vi "ADIS16448 Set Calibration Time.vi"(8 "error in (no error)":errorcluster, 10 "Calibration Time":T1, 11 "ADIS16448DevRef in":T2={"DevStatus"={"status"=FALSE, "code"=0, "source"=""}, "Hardware Config"={"SPI Clock Rate (Hz)"=1000000.0, "IMU SPI Mode (3)"=enum."Mode 3 (Clk Idle High,Sample on Trailing)", "IMU Reset Pin"=enum."SPI Port CS2", "IMU SPI Bus"=enum."SPI On-Board, CS0", "IMU Data Ready Pin"=enum."SPI Port CS1", "Stall Config"={"Pow2BytesPerRead"=255, "StallTicks"=640, "CsToSclkTicks"=5}, "IMU Status LED Pin"=enum."DIO MXP 9"}, "Calibration Complete"=refnum, "Status reference"=refnum, "Sychronous Process VI"=refnum, "Cmd FIFO"=refnum, "Source"={"DevStatus"={"status"=FALSE, "code"=0, "source"=""}, "AnalogTriggerMode?"=FALSE, "DigitalMode"={"DIO Channel"=enum."Disabled"}, "AnalogTriggerMode"={"AnalogTriggerIndex"=enum."Trig 0", "OutputType"=enum."InWindow"}}, "Data FIFO"=refnum, "IMU Status LED Pin"=enum."DIO MXP 9", "Calibration Time (ms)"=0, "Data Reference"=refnum}) -> (0 "error out":errorcluster, 3 "ADIS16448DevRef out":T2={"DevStatus"={"status"=FALSE, "code"=0, "source"=""}, "Hardware Config"={"SPI Clock Rate (Hz)"=1000000.0, "IMU SPI Mode (3)"=enum."Mode 3 (Clk Idle High,Sample on Trailing)", "IMU Reset Pin"=enum."SPI Port CS2", "IMU SPI Bus"=enum."SPI On-Board, CS0", "IMU Data Ready Pin"=enum."SPI Port CS1", "Stall Config"={"Pow2BytesPerRead"=255, "StallTicks"=640, "CsToSclkTicks"=5}, "IMU Status LED Pin"=enum."DIO MXP 9"}, "Calibration Complete"=refnum, "Status reference"=refnum, "Sychronous Process VI"=refnum, "Cmd FIFO"=refnum, "Source"={"DevStatus"={"status"=FALSE, "code"=0, "source"=""}, "AnalogTriggerMode?"=FALSE, "DigitalMode"={"DIO Channel"=enum."Disabled"}, "AnalogTriggerMode"={"AnalogTriggerIndex"=enum."Trig 0", "OutputType"=enum."InWindow"}}, "Data FIFO"=refnum, "IMU Status LED Pin"=enum."DIO MXP 9", "Calibration Time (ms)"=0, "Data Reference"=refnum})   [LabVIEW 2025]
doc: "This VI is deprecated. Use the input on the recalibrate VI instead."
uses:
  <vilib>/Rock Robotics/WPI/ThirdParty/ADI/ADIS16448/Typedef/ADIS16448 Command Type.ctl
  <vilib>/Rock Robotics/SystemInterfaces/DIO/FPGA_DIOChannel.ctl
  <vilib>/Rock Robotics/SystemInterfaces/spilib/spi_bus.ctl
  <vilib>/Rock Robotics/WPI/SPI/WPI_SPIMode.ctl
  <vilib>/Rock Robotics/WPI/ThirdParty/ADI/ADIS16448/Typedef/ADIS16448 Hardware Configuration.ctl
  <vilib>/Rock Robotics/WPI/ThirdParty/ADI/ADIS16448/Typedef/ADIS16448 Device Reference.ctl
  <vilib>/Rock Robotics/WPI/ThirdParty/ADI/ADIS16448/Typedef/ADIS16448 Data.ctl
  <vilib>/Rock Robotics/WPI/ThirdParty/ADI/ADIS16448/Typedef/ADIS16448 Status.ctl
  <vilib>/Rock Robotics/WPI/ThirdParty/ADI/ADIS16448/Typedef/ADIS16448 Process.ctl
  <vilib>/Rock Robotics/SystemInterfaces/DIO/FPGA_DIODigitalSourceChannel.ctl
  <vilib>/Rock Robotics/SystemInterfaces/AnalogTrigger/FPGA_AnalogTriggerIndex.ctl
  <vilib>/Rock Robotics/SystemInterfaces/AnalogTrigger/FPGA_AnalogTriggerOutType.ctl
  <vilib>/Rock Robotics/SystemInterfaces/CounterEncoderSourceConvertion/FPGA_CounterEncoderSourceConvertionLVSourceType.ctl
  <vilib>/Rock Robotics/WPI/ThirdParty/ADI/ADIS16448/Typedef/ADIS16448 Calibration Time.ctl
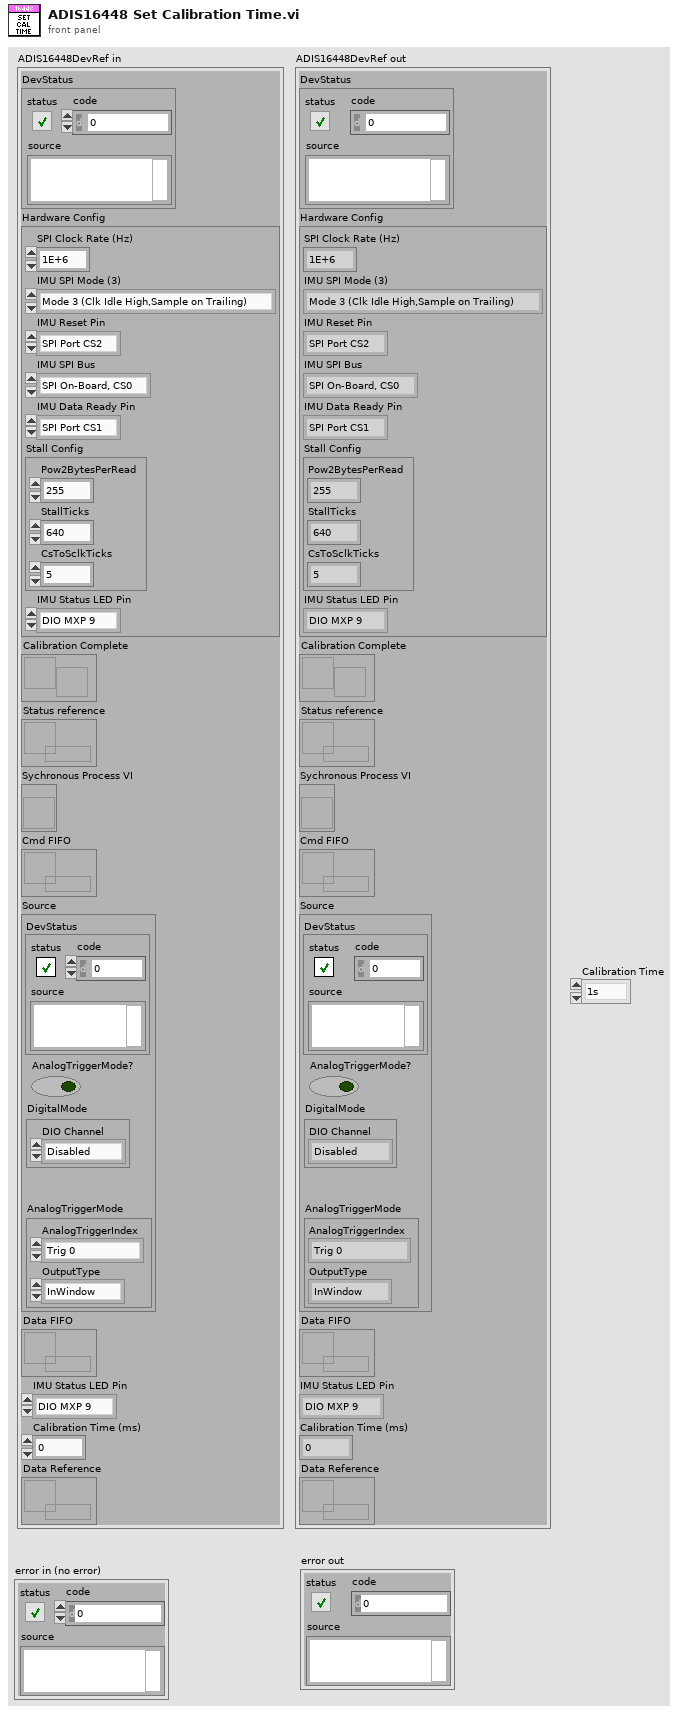
[diagram p1: front panel]
types:
  T1 = typedef "ADIS16448 Calibration Time.ctl" = enum16{"1s", "s", "4.9ms", "9.8ms", "19.5ms", "39.1ms", "78.1ms", "156.3ms", "312.5ms", "625ms", "1.25s", "2.5s", "5s", "10s", "20s", "40s", "80s", "160s", "320s"}
  T2 = typedef "ADIS16448 Device Reference.ctl" = cluster{"DevStatus":errorcluster, "Hardware Config":T3, "Calibration Complete":refnum<notifier>, "Status reference":refnum<data-value>, "Sychronous Process VI":T7, "Cmd FIFO":refnum<k33>, "Source":T8, "Data FIFO":refnum<k33>, "IMU Status LED Pin":T5, "Calibration Time (ms)":u32, "Data Reference":refnum<data-value>}
  T3 = typedef "ADIS16448 Hardware Configuration.ctl" = cluster{"SPI Clock Rate (Hz)":dbl, "IMU SPI Mode (3)":T4, "IMU Reset Pin":T5, "IMU SPI Bus":T6, "IMU Data Ready Pin":T5, "Stall Config":cluster{"Pow2BytesPerRead":u8, "StallTicks":u16, "CsToSclkTicks":u8}, "IMU Status LED Pin":T5}
  T4 = typedef "WPI_SPIMode.ctl" = enum16{"Mode 0 (Clk Idle Low,Sample on Leading)", "Mode 1 (Clk Idle Low,Sample on Trailing)", "Mode 2 (Clk Idle High,Sample on Leading)", "Mode 3 (Clk Idle High,Sample on Trailing)"}
  T5 = typedef "FPGA_DIOChannel.ctl" = enum8{"DIO 0", "DIO 1", "DIO 2", "DIO 3", "DIO 4", "DIO 5", "DIO 6", "DIO 7", "DIO 8", "DIO 9", "DIO MXP 0", "DIO MXP 1", "DIO MXP 2", "DIO MXP 3", "DIO MXP 4", "DIO MXP 5", "DIO MXP 6", "DIO MXP 7", "DIO MXP 8", "DIO MXP 9", "DIO MXP 10", "DIO MXP 11", "DIO MXP 12", "DIO MXP 13", "DIO MXP 14", "DIO MXP 15", "SPI Port CS1", "SPI Port CS2", "SPI Port CS3", "SPI Port MISO", "SPI Port MOSI", "Invalid"}
  T6 = typedef "spi_bus.ctl" = enum16{"SPI On-Board, CS0", "SPI On-Board, CS1", "SPI On-Board, CS2", "SPI On-Board, CS3", "SPI MXP", "Invalid"}
  T7 = typedef "ADIS16448 Process.ctl" = refnum<vi>
  T8 = typedef "FPGA_CounterEncoderSourceConvertionLVSourceType.ctl" = cluster{"DevStatus":errorcluster, "AnalogTriggerMode?":bool, "DigitalMode":cluster{"DIO Channel":T9}, "AnalogTriggerMode":cluster{"AnalogTriggerIndex":T10, "OutputType":T11}}
  T9 = typedef "FPGA_DIODigitalSourceChannel.ctl" = enum8{"DIO 0", "DIO 1", "DIO 2", "DIO 3", "DIO 4", "DIO 5", "DIO 6", "DIO 7", "DIO 8", "DIO 9", "DIO MXP 0", "DIO MXP 1", "DIO MXP 2", "DIO MXP 3", "DIO MXP 4", "DIO MXP 5", "DIO MXP 6", "DIO MXP 7", "DIO MXP 8", "DIO MXP 9", "DIO MXP 10", "DIO MXP 11", "DIO MXP 12", "DIO MXP 13", "DIO MXP 14", "DIO MXP 15", "SPI Port CS1", "SPI Port CS2", "SPI Port CS3", "SPI Port MISO", "SPI Port MOSI", "Disabled"}
  T10 = typedef "FPGA_AnalogTriggerIndex.ctl" = enum8{"Trig 0", "Trig 1", "Trig 2", "Trig 3", "Trig 4", "Trig 5", "Trig 6", "Trig 7", "Invalid"}
  T11 = typedef "FPGA_AnalogTriggerOutType.ctl" = enum16{"InWindow", "TriggerState", "Rising", "Falling"}
  T12 = typedef "ADIS16448 Command Type.ctl" = cluster{"Command":enum16{"None", "Reset", "Rewrite Config", "Start Recal", "Recalibrate", "Recal Complete", "Exit Auto SPI", "Start Auto SPI", "Configure Cal"}, "Data":u32}
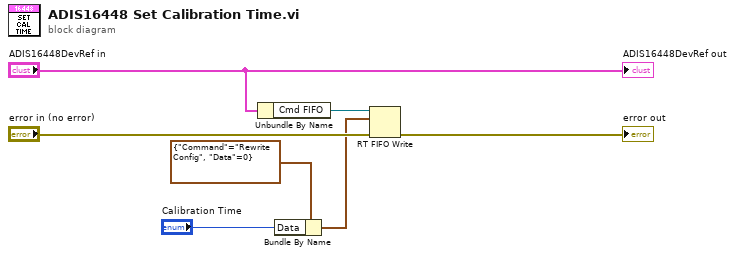
[diagram p0: block diagram]
diagram:
  n1 = Unbundle By Name("ADIS16448DevRef in") -> ("Cmd FIFO"=w7:refnum<k33>)
  n2 = Bundle By Name(cluster=T12 {"Command"=enum."Rewrite Config", "Data"=0} ("element"), "Data"="Calibration Time") -> (w1:T12)
  n3 = RT FIFO Write(0:w7, 1:w1, 3:"error in (no error)") -> (11:→"error out":errorcluster)  [unwired: 2 in, 3 out]
  "ADIS16448DevRef out" <- "ADIS16448DevRef in"
